vi "Write configuration.vi"(8 "error in":errorcluster, 10 "configuration":refnum<class "NISE_CEF_serializable configuration.lvclass">, 11 "cfg group in":refnum<class "cfg group.lvclass">) -> (0 "error out":errorcluster, 3 "cfg group out":refnum<class "cfg group.lvclass">)   [LabVIEW 2013, in "cfg group.lvclass"]
uses:
  cfg group.lvclass
  groupcfg/group configuration.lvclass
  CEF_TreeControl/serializable configuration/NISE_CEF_serializable configuration.lvclass
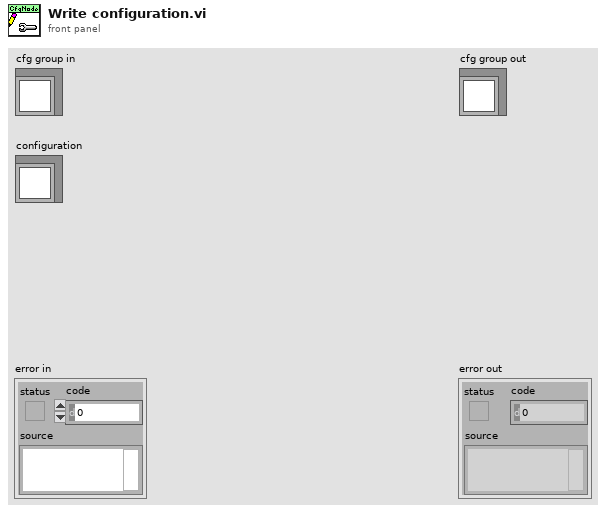
[diagram p1: front panel]
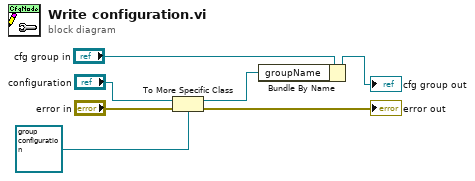
[diagram p0: block diagram]
diagram:
  n1 = To More Specific Class(target class=refnum<class "group configuration.lvclass"> refnum ("group configuration.lvclass"), reference="configuration", error in="error in") -> (specific class reference=w1:refnum<class "group configuration.lvclass">, error out=→"error out":errorcluster)
  n2 = Bundle By Name(cluster="cfg group in", "groupName"=w1) -> (→"cfg group out":refnum<class "cfg group.lvclass">)
